vi "StandAloneTransient_NIDCPOWER_PSU_POWER_ON_V1.vi"(8 "error in":errorcluster caption="error in (no error)", 9 "voltage level":dbl format="%.6p", 10 "channel name":string, 11 "resource name":refnum<k15>="PS_4110" caption="Hardware Force Reset") -> (0 "error out":errorcluster, 3 "current limit":dbl)   [LabVIEW 2019]
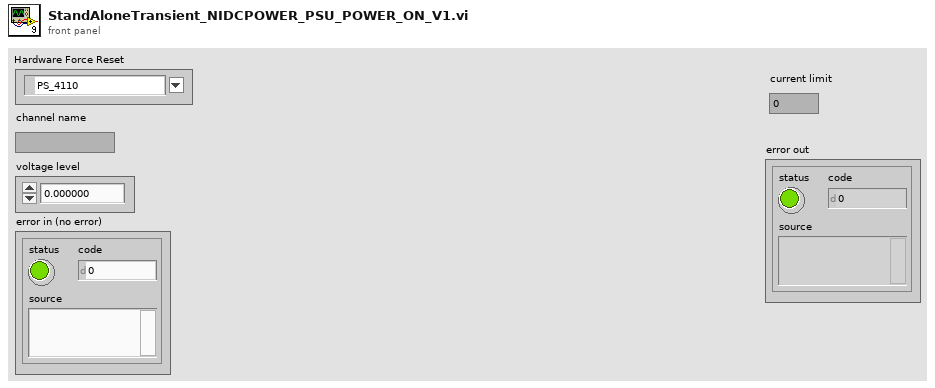
[diagram p1: front panel]
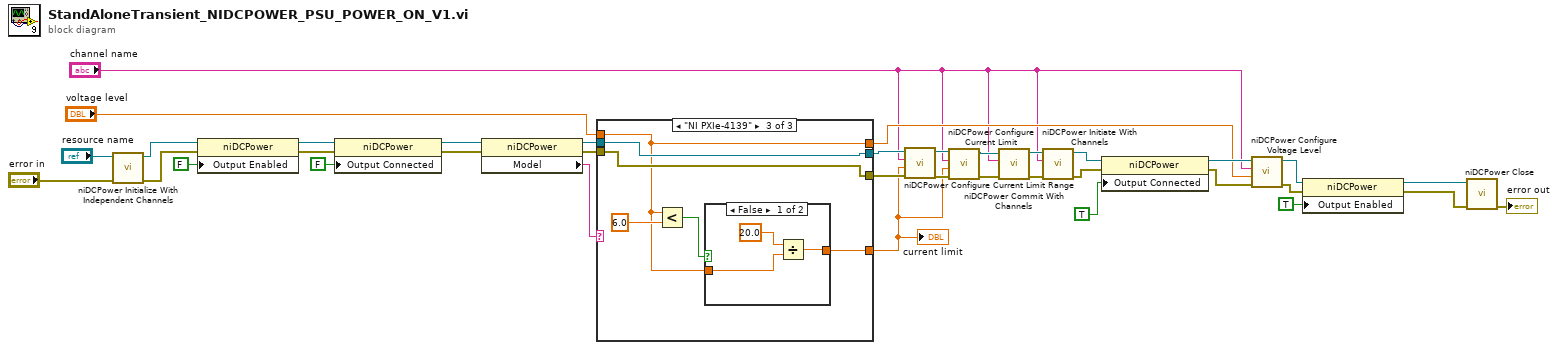
[diagram p0: block diagram]
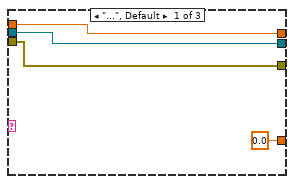
[diagram p2: hidden frame]
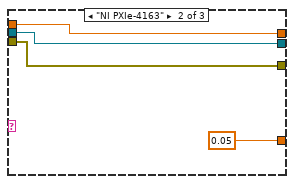
[diagram p3: hidden frame]
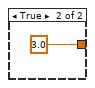
[diagram p4: hidden frame]
diagram:
  n1 = call <instrlib>:"niDCPower Initialize With Independent Channels.vi"("error in (no error)"="error in", "resource name"="resource name") -> ("error out"=w30:errorcluster, "instrument handle out"=w29:refnum<k15>)  [unwired: 8 in]
  n2 = property class="niDCPower"(reference=w29, error in=w30, "Output Enabled"=FALSE ("Source:Output Enabled")) -> (reference out=w32:refnum<k15>, error out=w31:errorcluster)
  n3 = property class="niDCPower"(reference=w32, error in=w31, "Output Connected"=FALSE ("Source:Output Connected")) -> (reference out=w10:refnum<k15>, error out=w11:errorcluster)
  n4 = property class="niDCPower"(reference=w10, error in=w11) -> (reference out=w4:refnum<k15>, error out=w5:errorcluster, "Model"=w9:string)
  n5 = case shown="\"NI PXIe-4139\"" w9 {
    tunnel: "voltage level" -> [w40 w42 w45]
    tunnel: [w40 w42 w45] -> w7
    tunnel: [w38 w44 w47] -> w6
    tunnel: w5 -> [w38 w44 w47]
    tunnel: w4 -> [w37 w43 w48]
    tunnel: [w37 w43 w48] -> w3
    tunnel: [0.0 ("current limit range") 0.05 ("current limit range") w46] -> w2
    frame "...", Default {
    }
    frame "NI PXIe-4163" {
    }
    frame "NI PXIe-4139" {
      n6 = Less?(x=w45, y=6.0) -> (x < y?=w49:bool)
      n7 = case shown="False" w49 {
        tunnel: [w51 3.0 ("current limit range")] -> w46
        tunnel: w45 -> [w52 _]
        frame False {
          n8 = Divide(x=20.0, y=w52) -> (x/y=w51:dbl)
        }
        frame True {
        }
      }
    }
  }
  "current limit" <- w2
  n9 = call <instrlib>:"niDCPower Configure Current Limit Range.vi"("error in (no error)"=w6, "current limit range"=w2, "channel name"="channel name", "instrument handle"=w3) -> ("error out"=w12:errorcluster, "instrument handle out"=w15:refnum<k15>)  [unwired: 6 in]
  n10 = call <instrlib>:"niDCPower Configure Current Limit.vi"("error in (no error)"=w12, "current limit"=w2, "channel name"="channel name", "instrument handle"=w15) -> ("error out"=w13:errorcluster, "instrument handle out"=w14:refnum<k15>)  [unwired: 6 in]
  n11 = call <instrlib>:"niDCPower Commit With Channels.vi"("error in (no error)"=w13, "channel name"="channel name", "instrument handle"=w14) -> ("error out"=w25:errorcluster, "instrument handle out"=w36:refnum<k15>)  [unwired: 7 in]
  n12 = call <instrlib>:"niDCPower Initiate With Channels.vi"("error in (no error)"=w25, "channel name"="channel name", "instrument handle"=w36) -> ("error out"=w26:errorcluster, "instrument handle out"=w27:refnum<k15>)  [unwired: 7 in]
  n13 = property class="niDCPower"(reference=w27, error in=w26, "Output Connected"=TRUE ("Source:Output Connected")) -> (reference out=w24:refnum<k15>, error out=w23:errorcluster)
  n14 = call <instrlib>:"niDCPower Configure Voltage Level.vi"("error in (no error)"=w23, "voltage level"=w7, "channel name"="channel name", "instrument handle"=w24) -> ("error out"=w21:errorcluster, "instrument handle out"=w20:refnum<k15>)  [unwired: 6 in]
  n15 = property class="niDCPower"(reference=w20, error in=w21, "Output Enabled"=TRUE ("Source:Output Enabled")) -> (reference out=w17:refnum<k15>, error out=w18:errorcluster)
  n16 = call <instrlib>:"niDCPower Close.vi"("error in (no error)"=w18, "instrument handle"=w17) -> ("error out"=→"error out":errorcluster)  [unwired: 9 in]
